vi "Does sequence exist.vi"(7 "Sequence name":string, 11 "error in (no error)":errorcluster) -> (8 "Sequence  exsists":bool, 15 "error out":errorcluster)   [LabVIEW 2011]
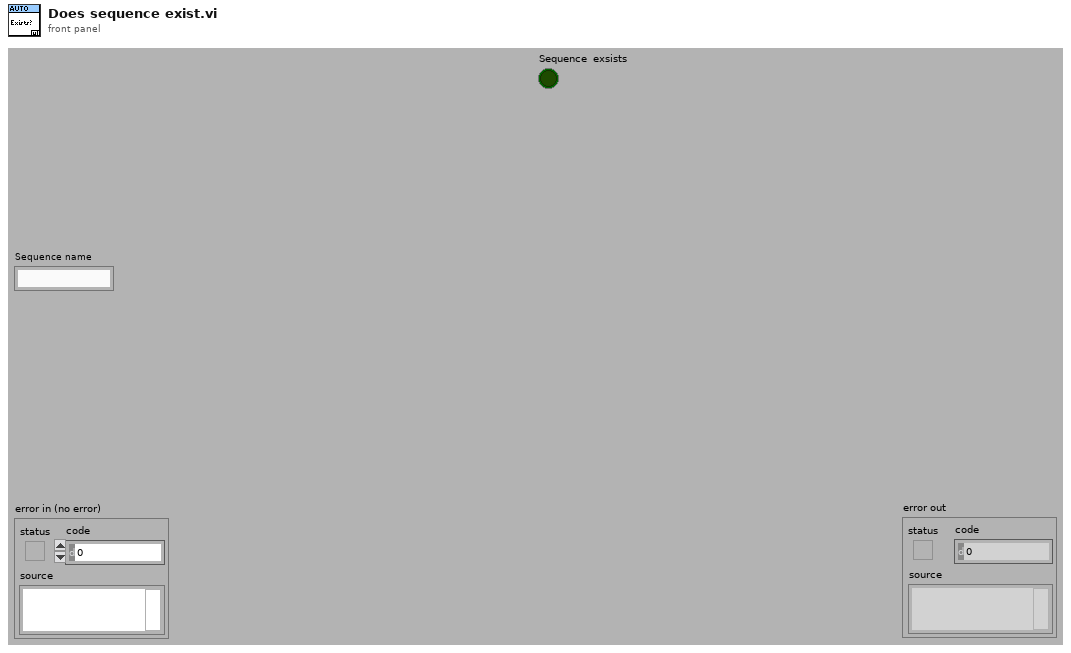
[diagram p1: front panel]
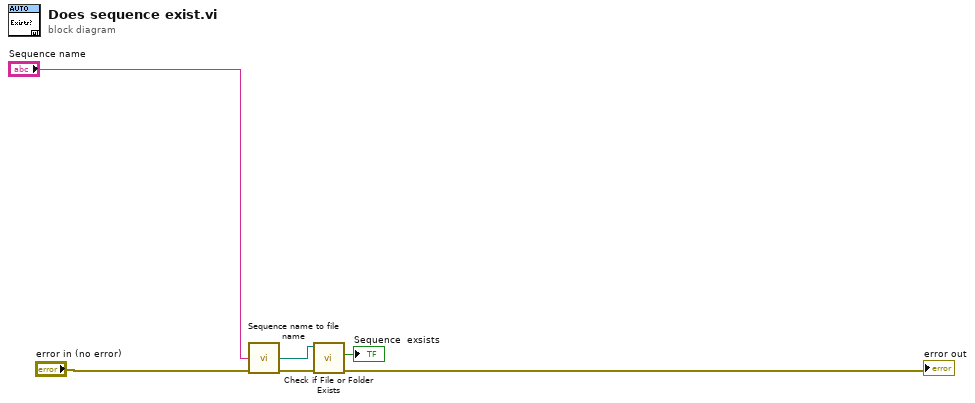
[diagram p0: block diagram]
diagram:
  n1 = call "Sequence name to file name.vi"("Sequence name"="Sequence name", "error in (no error)"="error in (no error)") -> ("Sequence file path"=w3:path, "error out"=w4:errorcluster)  [unwired: 12 in]
  n2 = call <vilib>:"Check if File or Folder Exists.vi"("error in (no error)"=w4, "path"=w3) -> ("error out"=→"error out":errorcluster, "file or folder exists?"=→"Sequence  exsists":bool)  [unwired: 7 in, 1 out]
